vi "Assign Locations.vi"(10 "error in (no error)":errorcluster, 11 "Picture In":refnum<class "Picture.lvclass">) -> (2 "error out":errorcluster, 3 "Picture Out":refnum<class "Picture.lvclass">)   [LabVIEW 2015, in "Picture.lvclass"]
uses:
  Picture.lvclass
  Picture.lvclass/Picture.ctl
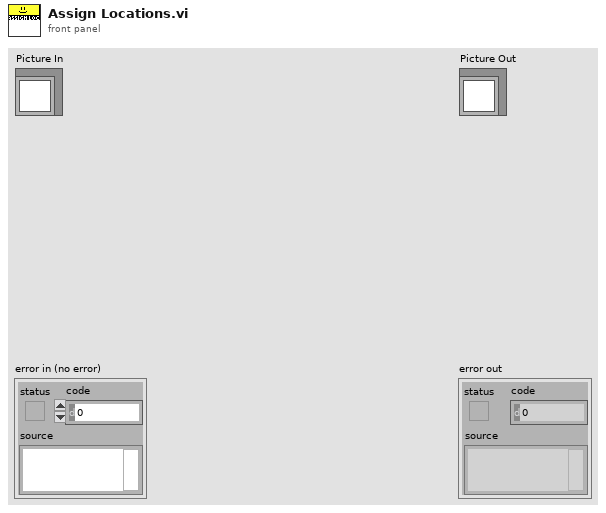
[diagram p1: front panel]
types:
  T1 = typedef "Common.lvlib/Position.ctl" = cluster{"Column":i32, "Row":i32}
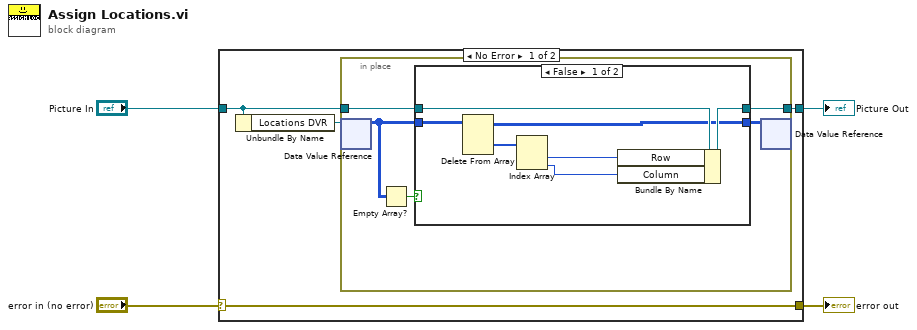
[diagram p0: block diagram]
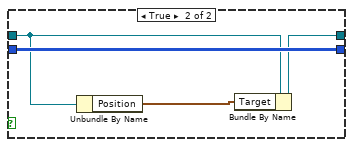
[diagram p2: hidden frame]
diagram:
  n1 = case shown="No Error" "error in (no error)" {
    selector: "error in (no error)" -> [w8 w26]
    tunnel: [w8 w26] -> w3
    tunnel: [w6 w25] -> w1
    tunnel: "Picture In" -> [w7 w25]
    frame No Error {
      n2 = Unbundle By Name(w7) -> ("Locations DVR"=w5:refnum<data-value>)
      n3 = in-place {
        in-place-border: w7 -> [w12]
        in-place-border: [w11] -> w6
        n4 = in-place-dvr #1(w5) -> (w10:i32[][])  [unwired: 1 out]
        n5 = Empty Array?(array=w10) -> (empty?=w13:bool)
        n6 = case shown="False" w13 {
          tunnel: w10 -> [w19 w24]
          tunnel: w12 -> [w20 w22]
          tunnel: [w17 w23] -> w11
          tunnel: [w14 w24] -> w9
          frame False {
            n7 = Delete From Array(array=w19) -> (deleted portion=w18:i32[], array with subset deleted=w14:i32[][])  [unwired: 3 in]
            n8 = Index Array(array=w18) -> (element #1=w16:i32, element #2=w15:i32)  [unwired: 2 in]
            n9 = Bundle By Name(cluster=w20, "Row"=w16, "Column"=w15) -> (w17:refnum<class "Picture.lvclass">)
          }
          frame True {
            n10 = Unbundle By Name(w22) -> ("Position"=w21:T1)
            n11 = Bundle By Name(cluster=w22, "Target"=w21) -> (w23:refnum<class "Picture.lvclass">)
          }
        }
        n12 = in-place-dvr #1(w9) -> ()  [unwired: 2 out]
      }
    }
    frame Error {
    }
  }
  "error out" <- w3
  "Picture Out" <- w1
